vi "File List Get file by index.vi"(10 "File index":i32, 11 "File List in":refnum<class "File List.lvclass">) -> (1 "Current file index out":i32, 2 "Current file out":path, 3 "File List out":refnum<class "File List.lvclass">)   [LabVIEW 2011, in "COSYLib.lvlib" / "File List.lvclass"]
doc: "Activates the file at a specific index in the list, and returns it.\nIf an invalid index is given, nothing is done, and an \"empty path\" and index \"-1\" are returned."
uses:
  File List.lvclass
  File List.lvclass/File List.ctl
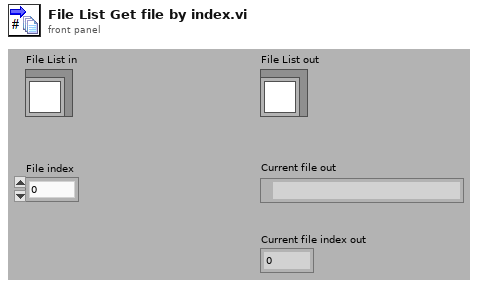
[diagram p1: front panel]
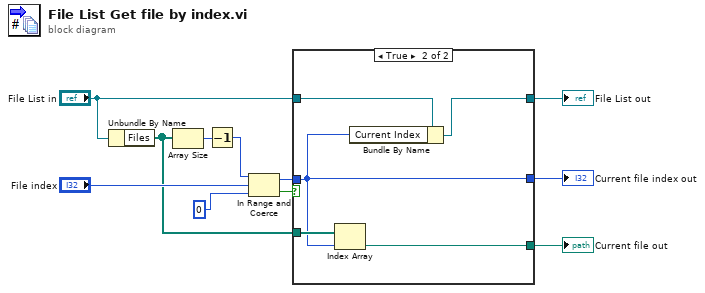
[diagram p0: block diagram]
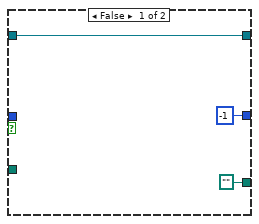
[diagram p2: hidden frame]
diagram:
  n1 = Unbundle By Name("File List in") -> ("Files"=w4:path[])
  n2 = Array Size(array=w4) -> (size(s)=w3:i32)
  n3 = Decrement(x=w3) -> (x-1=w2:i32)
  n4 = In Range and Coerce(upper limit=w2, x="File index", lower limit=0) -> (coerced(x)=w5:i32, In Range?=w9:bool)
  n5 = case shown="True" w9 {
    tunnel: "File List in" -> [w13 w19]
    tunnel: [w13 w18] -> w7
    tunnel: [path "" w16] -> w6
    tunnel: w5 -> [_ w15]
    tunnel: w4 -> [_ w17]
    tunnel: [-1 ("lower limit") w15] -> w1
    frame False {
    }
    frame True {
      n6 = Index Array(array=w17, index=w15) -> (element=w16:path)
      n7 = Bundle By Name(cluster=w19, "Current Index"=w15) -> (w18:refnum<class "File List.lvclass">)
    }
  }
  "File List out" <- w7
  "Current file out" <- w6
  "Current file index out" <- w1
